vi "Get Limits.vi"(0 "object in":refnum<class "HPS-17000-PowerModule.lvclass">, 11 "Error In":errorcluster) -> (4 "object out":refnum<class "HPS-17000-PowerModule.lvclass">, 6 "Limits":T1, 15 "Error Out":errorcluster)   [LabVIEW 2023, in "HPS-17000-PowerModule.lvlib" / "HPS-17000-PowerModule.lvclass"]
uses:
  HPS-17000-PowerModule.lvclass
  builds/PowerModuleInterface/home/lvuser/natinst/bin/PowerModuleInterface.lvlibp/Classes/PowerModule_interface/Limits.ctl
  <instrlib>/HPS-17000/Internal/Get Limits Multi.vi
  <instrlib>/HPS-17000/HPS-17000.lvclass
  builds/PowerModuleInterface/home/lvuser/natinst/bin/PowerModuleInterface.lvlibp/Classes/PowerModule_interface/PowerModuleInterface.lvclass
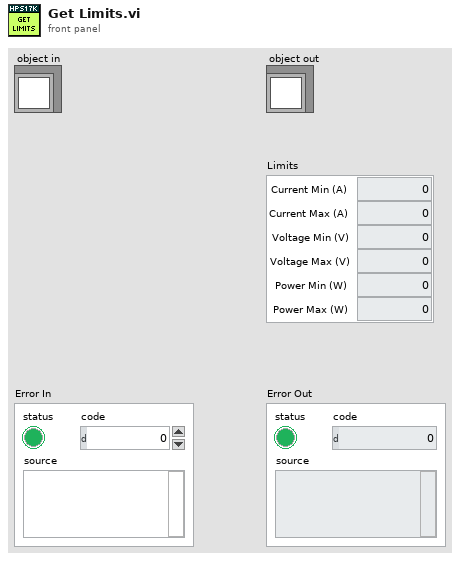
[diagram p1: front panel]
types:
  T1 = typedef "PowerModuleInterface.lvlibp/PowerModuleInterface.lvclass/Limits.ctl" = cluster{"Current Max (A)":dbl, "Current Min (A)":dbl, "Voltage Max (V)":dbl, "Voltage Min (V)":dbl, "Power Max (W)":dbl, "Power Min (W)":dbl}
  T2 = typedef "HPS-17000-PowerModule.lvlib/HPS-17000-PowerModule.lvclass/ObjectAttributes.ctl" = cluster{"JSON Config Path":path, "Configuration":T3, "GM ID":string, "HPS17000 Refs":refnum<class "HPS-17000.lvclass">[], "connected":bool, "reserved":bool, "events":T5, "nibatterycycler_grpc_Setpoint":T6, "last timestamp":i64, "mode":T7, "range":T8, "measurement array":T9[]}
  T3 = typedef "HPS-17000-PowerModule.lvlib/HPS-17000-PowerModule.lvclass/Configuration.ctl" = cluster{"TSN NIC IP Address":string, "HPS17000 IP Addresses":string[], "HPS Topology":enum16{"SINGLE", "MULTI"}, "Setpoint Stream Config":T4, "Measurement Array Size":i32}
  T4 = typedef "Cycler.lvclass/Setpoint Stream Basic Config.ctl" = cluster{"local address":string, "receiver port":u16}
  T5 = typedef "HPS-17000.lvclass/Multi-Cycler Events.ctl" = cluster{"heartbeats events":refnum<user-event>[], "faults events":refnum<user-event>[], "network sync event":refnum<user-event>[], "setpoint status event":refnum<user-event>[]}
  T6 = typedef "NI_BC_client.lvlib/nibatterycycler_grpc_Setpoint.ctl" = cluster{"voltage":sgl, "current":sgl, "min_power":sgl, "max_power":sgl, "resistance":sgl}
  T7 = typedef "HPS-17000-PowerModule.lvlib/HPS-17000-PowerModule.lvclass/Mode.ctl" = u16
  T8 = typedef "PowerModuleInterface.lvlibp/PowerModuleInterface.lvclass/Range.ctl" = cluster{"Current Max (A)":dbl, "Current Min (A)":dbl, "Voltage Max (V)":dbl, "Voltage Min (V)":dbl}
  T9 = typedef "PowerModuleInterface.lvlibp/PowerModuleInterface.lvclass/Measurements.ctl" = cluster{"measured voltage (V)":dbl, "measured current (A)":dbl, "setpoint voltage (V)":dbl, "setpoint current (A)":dbl, "timestamp":dbl}
  T10 = typedef "HPS-17000.lvclass/Limits.ctl" = cluster{"Current Max Limit":sgl, "Current Min Limit":sgl, "Voltage Max Limit":sgl, "Voltage Min Limit":sgl, "Power Max Limit":sgl, "Power Min Limit":sgl}
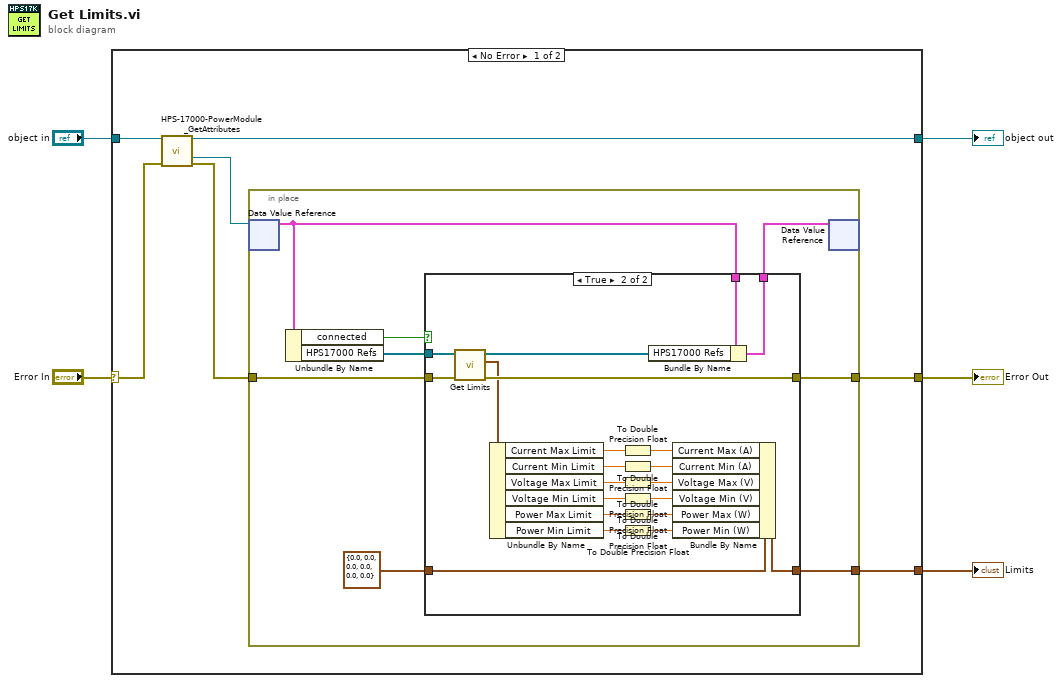
[diagram p0: block diagram]
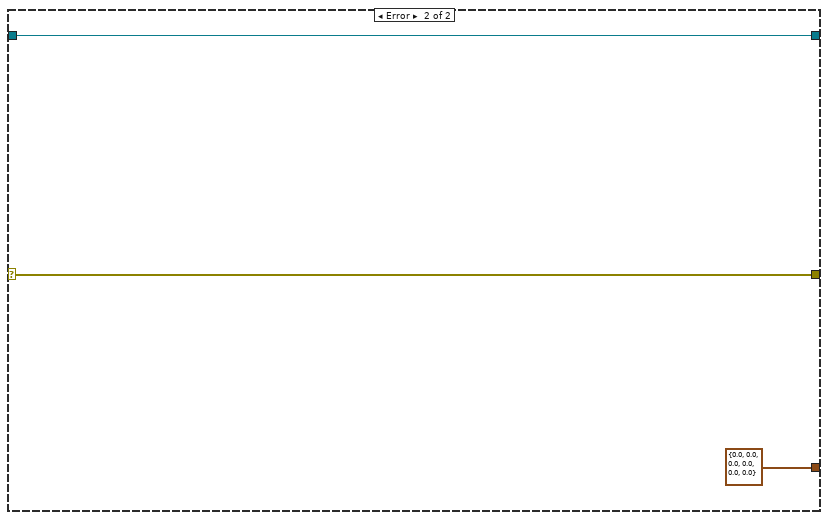
[diagram p3: hidden frame]
diagram:
  n1 = case shown="No Error" "Error In" {
    selector: "Error In" -> [w11 w46]
    tunnel: "object in" -> [w12 w47]
    tunnel: [w7 w47] -> w4
    tunnel: [w8 w46] -> w2
    tunnel: [w6 T1 {"Current Max (A)"=0.0, "Current Min (A)"=0.0, "Voltage Max (V)"=0.0, "Voltage Min (V)"=0.0, "Power Max (W)"=0.0, "Power Min (W)"=0.0} ("Limits")] -> w1
    frame No Error {
      n2 = call "HPS-17000-PowerModule_GetAttributes.vi"("reference in"=w12, "Error In"=w11) -> ("reference out"=w7:refnum<class "HPS-17000-PowerModule.lvclass">, "DataRef"=w10:refnum<data-value>, "Error Out"=w9:errorcluster)  [unwired: 10 in, 1 out]
      n3 = in-place {
        in-place-border: w9 -> [w18]
        in-place-border: [w17] -> w8
        in-place-border: [w14] -> w6
        n4 = in-place-dvr #1(w10) -> (w19:T2)  [unwired: 1 out]
        n5 = Unbundle By Name(w19) -> ("connected"=w15:bool, "HPS17000 Refs"=w16:refnum<class "HPS-17000.lvclass">[])
        n6 = case shown="True" w15 {
          tunnel: [w23 w44] -> w20
          tunnel: w19 -> [w23 w43]
          tunnel: w18 -> [w22 w40]
          tunnel: [w22 w39] -> w17
          tunnel: w16 -> [_ w42]
          tunnel: [w21 w38] -> w14
          tunnel: T1 {"Current Max (A)"=0.0, "Current Min (A)"=0.0, "Voltage Max (V)"=0.0, "Voltage Min (V)"=0.0, "Power Max (W)"=0.0, "Power Min (W)"=0.0} ("Limits") -> [w21 w24]
          frame False {
          }
          frame True {
            n7 = call-poly <instrlib>:"Get Limits.vi"("error in"=w40, "cycler refs in"=w42) -> ("error out"=w39:errorcluster, "limits out"=w37:T10, "cycler refs out"=w41:refnum<class "HPS-17000.lvclass">[])  [unwired: 7 in]
            n8 = Unbundle By Name(w37) -> ("Current Max Limit"=w26:sgl, "Current Min Limit"=w28:sgl, "Voltage Max Limit"=w30:sgl, "Voltage Min Limit"=w32:sgl, "Power Max Limit"=w34:sgl, "Power Min Limit"=w36:sgl)
            n9 = To Double Precision Float(number=w26) -> (double precision float=w25:dbl)
            n10 = To Double Precision Float(number=w28) -> (double precision float=w27:dbl)
            n11 = To Double Precision Float(number=w30) -> (double precision float=w29:dbl)
            n12 = To Double Precision Float(number=w32) -> (double precision float=w31:dbl)
            n13 = To Double Precision Float(number=w34) -> (double precision float=w33:dbl)
            n14 = To Double Precision Float(number=w36) -> (double precision float=w35:dbl)
            n15 = Bundle By Name(cluster=w43, "HPS17000 Refs"=w41) -> (w44:T2)
            n16 = Bundle By Name(cluster=w24, "Current Max (A)"=w25, "Current Min (A)"=w27, "Voltage Max (V)"=w29, "Voltage Min (V)"=w31, "Power Max (W)"=w33, "Power Min (W)"=w35) -> (w38:T1)
          }
        }
        n17 = in-place-dvr #1(w20) -> ()  [unwired: 2 out]
      }
    }
    frame Error {
    }
  }
  "Error Out" <- w2
  "object out" <- w4
  "Limits" <- w1
